vi "COMI Load Count.vi"(9 "load_value":u16, 10 "ch":i32, 11 "hDevice":u32) -> (3 "hDevice out":u32)   [LabVIEW 2017, in "Comidll.lvlib"]
doc: "void (COMI_LoadCount) (HANDLE hDevice, int ch, unsigned short load_value);"
uses:
  <userlib>/Comidll/Comidll.lvlib
  <userlib>/Comidll/Comidll.dll
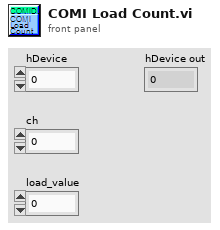
[diagram p1: front panel]
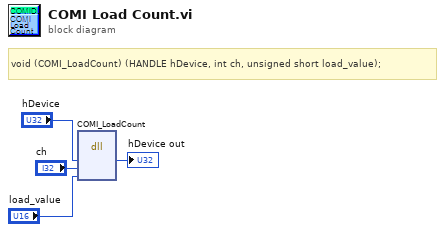
[diagram p0: block diagram]
diagram:
  # "void\t(COMI_LoadCount) (HANDLE hDevice, int ch, unsigned short load_value);"
  n1 = dll-call lib="C:/Program Files/National Instruments/LabVIEW 2017/user.lib/Comidll/Comidll.*" fn="COMI_LoadCount"("hDevice"="hDevice", "ch"="ch", "load_value"="load_value") -> ("hDevice"=→"hDevice out":u32)  [unwired: 6 in, 2 out]
